vi "OC2 Setup Sensor.vi"(4 "Enable":bool, 5 "error in (no error)":errorcluster, 6 "sensor report in":T1 {"Averaging" items=["Off", "On"]; "Unit" items=["deg C", "deg F", "deg K"]; "C coeff." format="%.2f"; "X coeff." format="%.2f"; "X2 coeff." format="%.2f"; "Sensor" items=["None", "PT100", "LM35", "LM50", "LM51", "LM60", "LM61", "Other"]}, 7 "VISA resource name":refnum<visa-resource-name>) -> (0 "error out":errorcluster, 1 "sensor report out":T1 {"Averaging" items=["Off", "On"]; "Unit" items=["deg C", "deg F", "deg K"]; "C coeff." format="%.2f"; "X coeff." format="%.2f"; "X2 coeff." format="%.2f"; "Sensor" items=["None", "PT100", "LM35", "LM50", "LM51", "LM60", "LM61", "Other"]}, 3 "dup VISA resource name":refnum<visa-resource-name>)   [LabVIEW 2009]
doc: "TCM Setup Sensor.vi\n\nVI that sets the sensor information, accepts a cluster that contains the following variables:\nSensor type - PT100, LM35 etc\nx2, x, c coefficients - quadratic equation information\nUnit - unit of measure degrees c, f and kelvin\nAveraging - off no averaging of the signal, on signal is averaged\n\n\nCOPYRIGHT ELECTRON DYNAMICS LTD"
panel:
  out "command data":string
  # "Set sensor variables"
  # "V1.02"
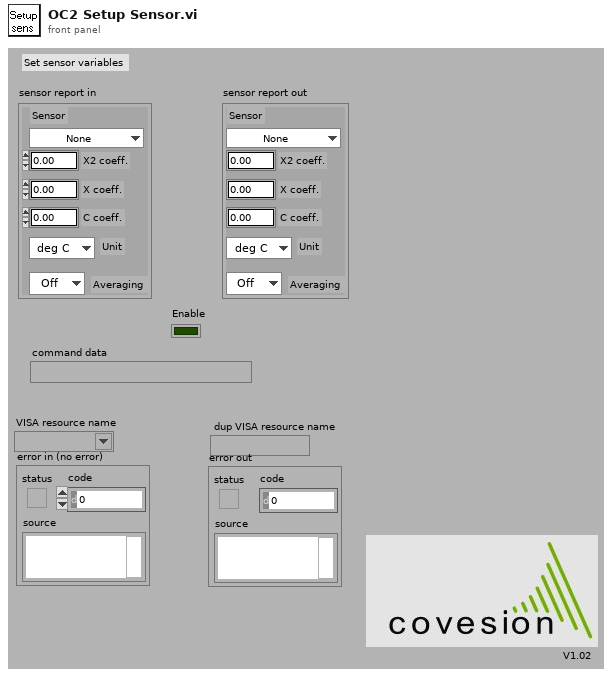
[diagram p1: front panel]
types:
  T1 = cluster{"Sensor":u16, "X2 coeff.":dbl, "X coeff.":dbl, "C coeff.":dbl, "Unit":u16, "Averaging":u16}
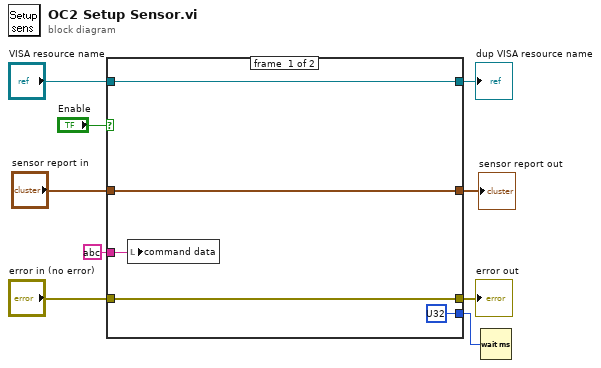
[diagram p0: block diagram]
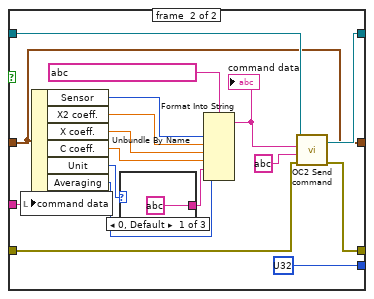
[diagram p2: hidden frame]
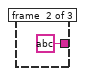
[diagram p3: hidden frame]
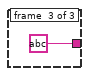
[diagram p4: hidden frame]
diagram:
  n1 = case shown="True" "Enable" {
    tunnel: "VISA resource name" -> [w14 w27]
    tunnel: [w14 w26] -> w8
    tunnel: "error in (no error)" -> [w13 w25]
    tunnel: [w13 w24] -> w6
    tunnel: "sensor report in" -> [w12 w17]
    tunnel: [w12 w17] -> w3
    tunnel: string ? -> [w11 w16]
    tunnel: [u32 ? ("milliseconds to wait") u32 ? ("milliseconds to wait")] -> w1
    frame #0 {
      n2 = local write "command data"(w11) -> ()
    }
    frame #1 {
      n3 = local write "command data"(w16) -> ()
      n4 = Unbundle By Name(w17) -> ("Sensor"=w23:u16, "X2 coeff."=w22:dbl, "X coeff."=w21:dbl, "C coeff."=w20:dbl, "Unit"=w19:u16, "Averaging"=w18:u16)
      n5 = case shown="0, Default" w19 {
        tunnel: [string ? string ? string ?] -> w28
        frame #0 {
        }
        frame #1 {
        }
        frame #2 {
        }
      }
      n6 = Format Into String(format string=string ?, w23, w22, w21, w20, w28, w18) -> (resulting string=w29:string)  [unwired: 2 in, 1 out]
      "command data" <- w29
      n7 = call "OC2 Send command.vi"("VISA resource name"=w27, "Command data"=w29, "Command"=string ?, "error in (no error)"=w25) -> ("dup VISA resource name"=w26:refnum<visa-resource-name>, "error out"=w24:errorcluster)  [unwired: 1 in]
    }
  }
  "dup VISA resource name" <- w8
  "error out" <- w6
  "sensor report out" <- w3
  n8 = Wait (ms)(milliseconds to wait=w1) -> ()  [unwired: 1 out]
